vi "CCD Example.vi"   [LabVIEW 2023]
uses:
  Source/Classes/CCD/CCD.lvclass
  Source/Libraries/DeviceManager/DeviceManager.lvlib
types:
  T1 = typedef "DeviceManager.lvlib/Broadcast Events--cluster.ctl" = cluster{"Module Did Init":refnum<user-event>, "Status Updated":refnum<user-event>, "Error Reported":refnum<user-event>, "Module Did Stop":refnum<user-event>, "Update Module Execution Status":refnum<user-event>}
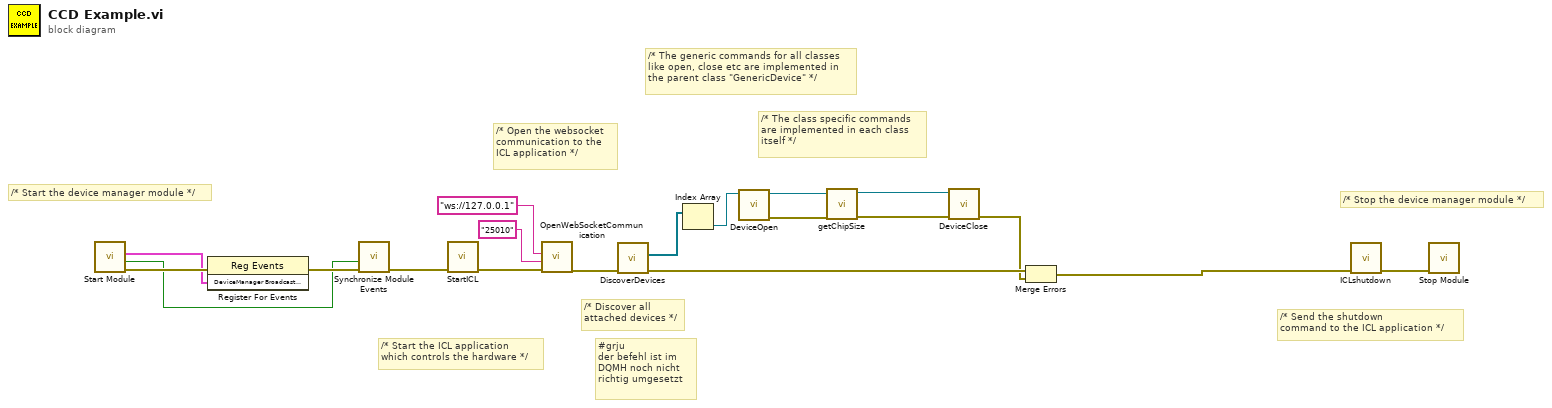
[diagram p0: block diagram]
diagram:
  # "#grju\nder befehl ist im\nDQMH noch nicht\nrichtig umgesetzt"
  # "/* Stop the device manager module */"
  # "/* Send the shutdown\ncommand to the ICL application */"
  # "/* The class specific commands\nare implemented in each class\nitself */"
  # "/* The generic commands for all classes\nlike open, close etc are implemented in\nthe parent class \"GenericDevice\" */"
  # "/* Discover all\nattached devices */"
  # "/* Open the websocket\ncommunication to the \nICL application */"
  # "/* Start the ICL application\nwhich controls the hardware */"
  # "/* Start the device manager module */"
  n1 = call "Start Module.vi"() -> ("error out"=w19:errorcluster, "Wait for Event Sync?"=w16:bool, "DeviceManager Broadcast Events"=w18:T1)  [unwired: 8 in, 1 out]
  n2 = register-events(error in=w19, w18) -> (error out=w17:errorcluster)  [unwired: 1 in, 1 out]
  n3 = call "Synchronize Module Events.vi"("error in"=w17, "Wait for Event Sync?"=w16) -> ("error out"=w15:errorcluster)  [unwired: 9 in]
  n4 = call "StartICL.vi"("error in"=w15) -> ("error out"=w14:errorcluster)  [unwired: 10 in]
  n5 = call "OpenWebSocketCommunication.vi"("error in"=w14, "WS Server Port"="25010", "WS Server IP"="ws://127.0.0.1") -> ("error out"=w11:errorcluster)  [unwired: 6 in, 2 out]
  n6 = call "DiscoverDevices.vi"("error in"=w11) -> ("error out"=w10:errorcluster, "CCDs"=w8:refnum<class "CCD.lvclass">[])  [unwired: 6 in, 3 out]
  n7 = Index Array(array=w8) -> (element=w7:refnum<class "CCD.lvclass">)  [unwired: 1 in]
  n8 = call-dynamic "DeviceOpen.vi"("GenericDevice in"=w7) -> ("error out"=w5:errorcluster, "GenericDevice out"=w6:refnum<class "CCD.lvclass">)  [unwired: 9 in]
  n9 = call-dynamic "getChipSize.vi"("error in (no error)"=w5, "CCD in"=w6) -> ("error out"=w4:errorcluster, "CCD out"=w3:refnum<class "CCD.lvclass">)  [unwired: 7 in, 1 out]
  n10 = call-dynamic "DeviceClose.vi"("error in (no error)"=w4, "GenericDevice in"=w3) -> ("error out"=w1:errorcluster)  [unwired: 8 in, 1 out]
  n11 = Merge Errors(w10, w1) -> (w2:errorcluster)
  n12 = call "ICLshutdown.vi"("error in"=w2) -> ("error out"=w9:errorcluster)  [unwired: 10 in]
  n13 = call "Stop Module.vi"("error in"=w9) -> ()  [unwired: 10 in, 1 out]
